vi "MSP6715-Control.vi"() -> ()   [LabVIEW 2015, in "MSP6715.lvlib"]
uses:
  MSP6715.lvlib
  <vilib>/Instr/_visa.llb/VISA Configure Serial Port (Instr).vi
panel:
  in  "参数值":dbl
  in  "命令字":T1(ring)
  in  "MyIndex":u8
  in  "等待时间(毫秒)":u32=100
  out "VISA":refnum<visa-resource-name>
  out "error out":errorcluster
  in  "error in":errorcluster caption="错误输入（无错误）"
  out "电压，电流，功率数组":dbl[](array[numeric])
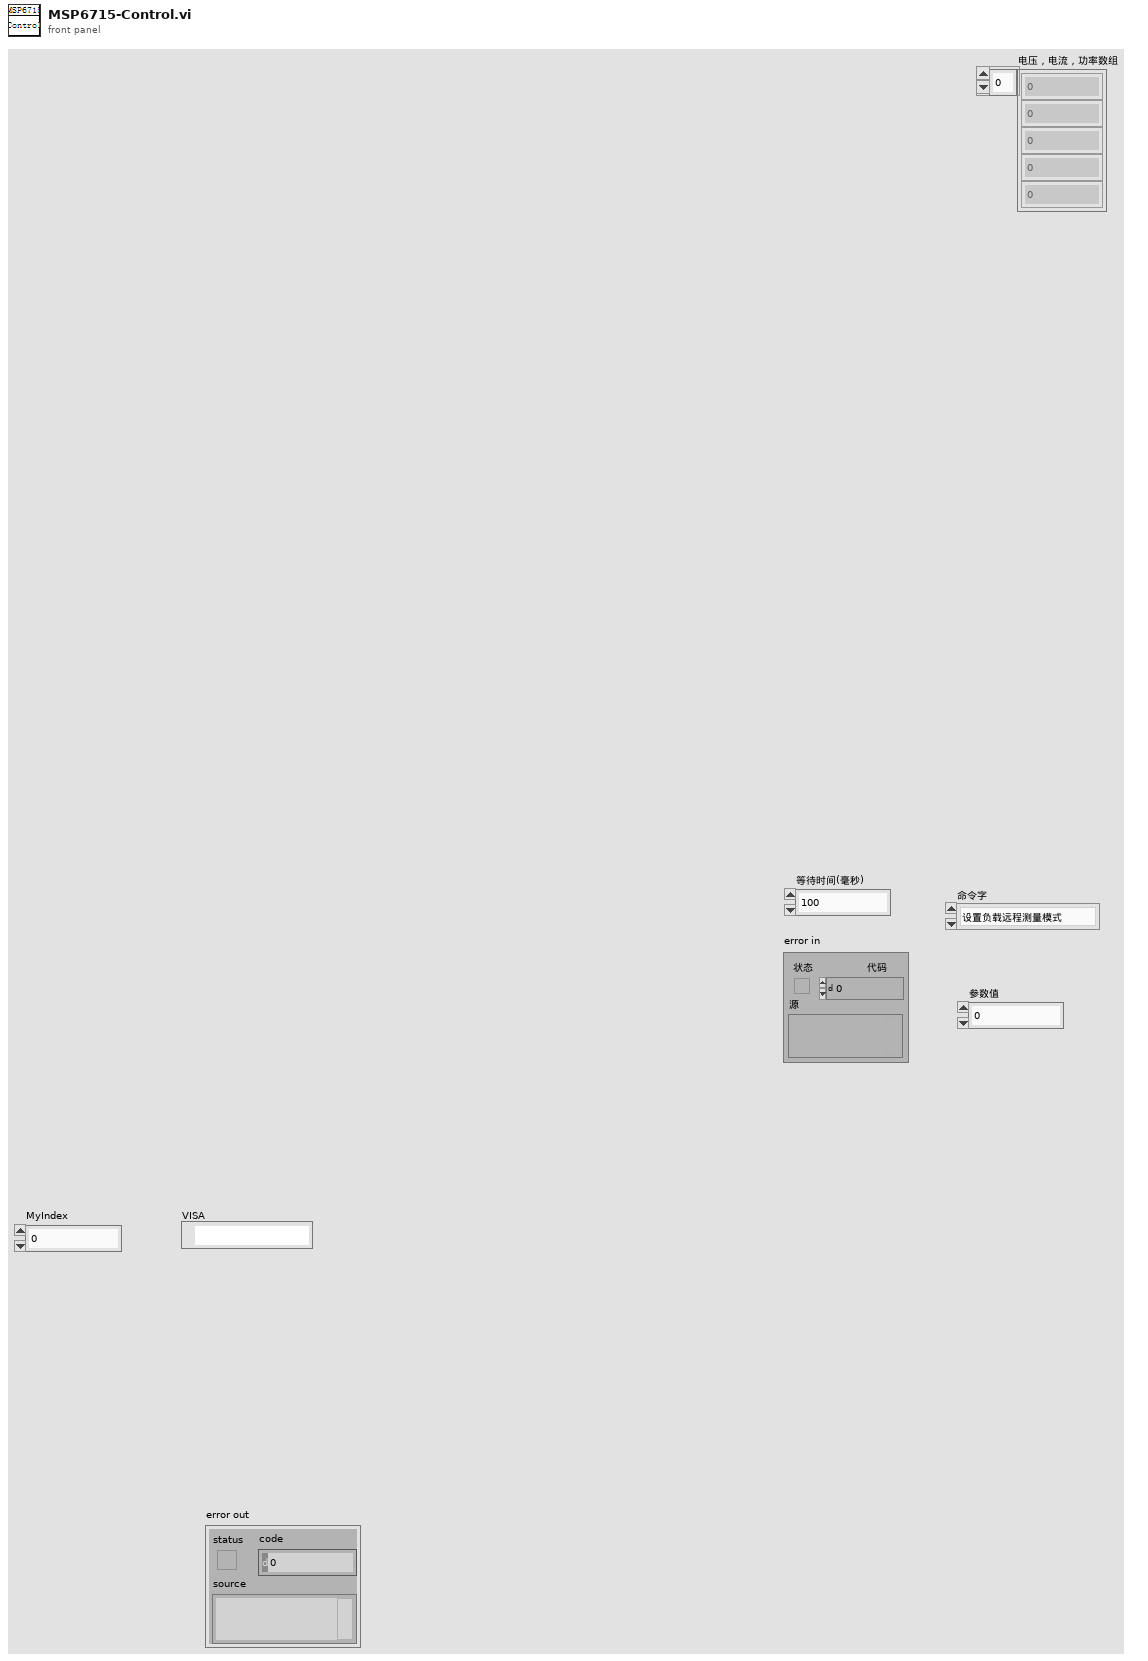
[diagram p1: front panel]
types:
  T1 = enum16{"设置负载远程测量模式", "读取负载的输入电压，电流，工率", "设置负载工作模式", "设置负载模式", "设置定电流值", "设置定电压值"}
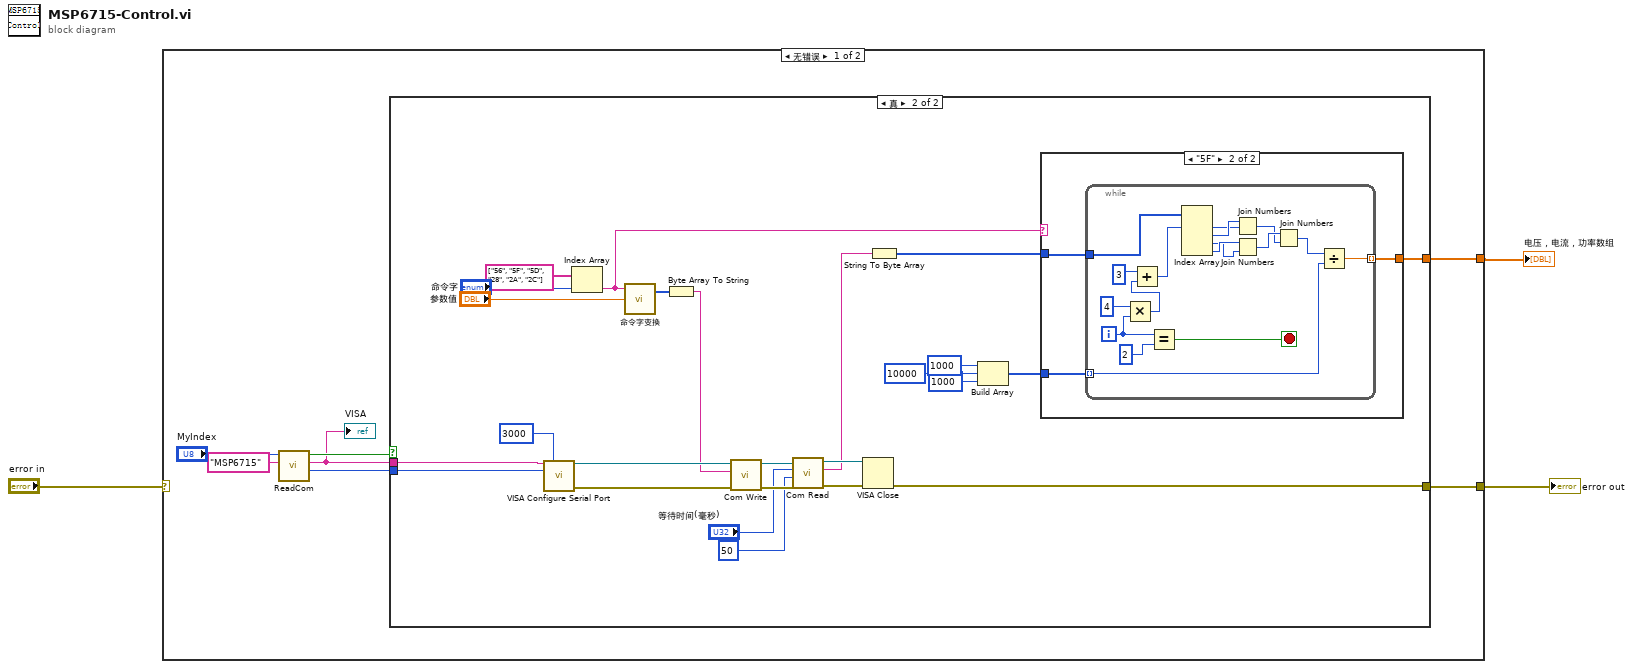
[diagram p0: block diagram]
diagram:
  n1 = case shown="无错误" "error in" {
    selector: "error in" -> [_ w56]
    tunnel: [w10 w56] -> w3
    tunnel: [w4 _] -> w1
    frame No Error {
      n2 = call "ReadCom.vi"("仪器名称"="MSP6715", "MyIndex"="MyIndex") -> ("Baudrate"=w5:i32, "COM"=w6:string, "OK?"=w7:bool)  [unwired: 7 in]
      "VISA" <- w6
      n3 = case shown="真" w7 {
        tunnel: [_ w35] -> w10
        tunnel: w6 -> [_ w34]
        tunnel: w5 -> [_ w33]
        tunnel: [_ w11] -> w4
        frame False {
        }
        frame True {
          n4 = call-poly "VISA Configure Serial Port"("VISA resource name"=w34, "timeout (10sec)"=u32 3000, "baud rate (9600)"=w33) -> ("VISA resource name out"=w31:refnum<visa-resource-name>, "error out"=w30:errorcluster)  [unwired: 11 in]
          n5 = Index Array(array=string[] ["56", "5F", "5D", "28", "2A", "2C"], index="命令字") -> (element=w12:string)
          n6 = call "命令字变换.vi"("命令字参数"="参数值", "命令字"=w12) -> ("Hex指令"=w20:u32[])  [unwired: 1 in, 1 out]
          n7 = Byte Array To String(unsigned byte array=w20) -> (string=w19:string)
          n8 = call "Com Write.vi"("错误输入（无错误）"=w30, "Wbuff"=w19, "VISA In"=w31) -> ("错误输出"=w28:errorcluster, "VISA Out"=w29:refnum<visa-resource-name>)  [unwired: 7 in]
          n9 = call "Com Read.vi"("错误输入（无错误）"=w28, "num"=u32 50, "超时"="等待时间(毫秒)", "VISA In"=w29) -> ("错误输出"=w27:errorcluster, "buff"=w18:string, "VISA Out"=w26:refnum<visa-resource-name>)  [unwired: 5 in]
          n10 = VISA Close(VISA resource name=w26, error in (no error)=w27) -> (error out=w35:errorcluster)
          n11 = String To Byte Array(string=w18) -> (unsigned byte array=w13:u8[])
          n12 = Build Array(1000, 10000, 1000) -> (w17:i32[])
          n13 = case shown="\"5F\"" w12 {
            tunnel: w13 -> [_ w38]
            tunnel: [_ w37] -> w11
            tunnel: w17 -> [_ w36]
            frame "假", Default {
            }
            frame "5F" {
              n14 = while {
                tunnel: w38 -> [w55]
                tunnel: [w44] -> w37 mode=indexing
                tunnel: w36 -> [w45] mode=indexing
                i -> [w41]
                stop <- w47 stop-if-true
                n15 = Multiply(x=4, y=w41) -> (x*y=w39:i32)
                n16 = Add(x=3, y=w39) -> (x+y=w43:i32)
                n17 = Equal?(x=w41, y=2) -> (x = y?=w47:bool)
                n18 = Index Array(array=w55, index #1=w43) -> (element #1=w51:u8, element #2=w52:u8, element #3=w53:u8, element #4=w54:u8)  [unwired: 3 in]
                n19 = Join Numbers(hi=w52, lo=w51) -> ((hi.lo)=w49:u16)
                n20 = Join Numbers(hi=w54, lo=w53) -> ((hi.lo)=w50:u16)
                n21 = Join Numbers(hi=w50, lo=w49) -> ((hi.lo)=w46:u32)
                n22 = Divide(x=w46, y=w45) -> (x/y=w44:dbl)
              }
            }
          }
        }
      }
    }
    frame Error {
    }
  }
  "电压，电流，功率数组" <- w1
  "error out" <- w3
